vi "GluePattern_Test(SubVI).vi"() -> ()   [LabVIEW 2016]
uses:
  C:/Users/Aerotech/Documents/BNL_ThermomechanicalStave/AerotechLibraries/Bin/Aerotech.A3200.dll
  AerotechLibraries/Bin/Aerotech.A3200.dll
  <vilib>/LabVIEW Interface for Arduino/Type Defs/Arduino Resource.ctl
  <vilib>/LabVIEW Interface for Arduino/Type Defs/Board Type.ctl
  <vilib>/LabVIEW Interface for Arduino/Type Defs/Pin Mode.ctl
  <vilib>/Utility/file.llb/Read Delimited Spreadsheet (DBL).vi
  <vilib>/LabVIEW Interface for Arduino/LabVIEW Interface for Arduino.lvlib
panel:
  out "DX [mm]":dbl=4.166666666666667
  out "DY [mm]":dbl=100.0
  in  "Type of Pattern":u16(ring) items=["Dots", "Lines"]
  out "Arduino Resource":T1={"VISA resource"="COM3", "Board Type"=enum."Uno", "Connection Type"=enum."USB / Serial", "Bytes Per Packet (15)"=15}
  in  "Digital I/O Pin":u8=7
  in  "Final Z":dbl=49.0
  out "Final Position":T3={"Final X"=45.83348650187174, "Final Y"=-0.00047053123122535695, "Final Z"=43.999513057466004}
  out "Column":i32=11
  out "Row":i32
  out "error out":errorcluster={"status"=FALSE, "code"=1073676294, "source"="VISA Read in LabVIEW Interface for Arduino.lvlib:Send Receive.vi->LabVIEW Interface for Arduino.lvlib:Digital Write Pin.vi->GluePattern_Test(SubVI).vi"}
  in  "Home?":bool
  out "XYZ Stage Control":refnum<k24>
  in  "File to be processed- Dots":path=path "C:/Users/Aerotech/Documents/BNL_ThermomechanicalStave/1_ModulePlacement/1_GluePatterning/LabVIEW_gluepattern_arraytest.csv"
  in  "Axis Speeds":T4={"vX [mm]"=15.0, "vY [mm]"=15.0, "vZ [mm] "=15.0}
  in  "Go to \ncoordinates":T5={"X [mm]"=0.0, "Y [mm]"=0.0, "Z [mm] "=44.0}
  out "DX[s]":dbl=0.2777777777777778 format="%#_2g"
  out "DY [s]":dbl=6.666666666666667 format="%#_2g"
  in  "Module width [mm]":dbl=50.0
  in  "Module length [mm]":dbl=100.0
  out "INPUT : Dot":bool[][](array[boolean])=[[TRUE, FALSE, TRUE, FALSE, TRUE, FALSE, TRUE, FALSE, TRUE, FALSE, TRUE, FALSE]]
  in  "Duration of glue \ndispensing [s]":dbl=0.25
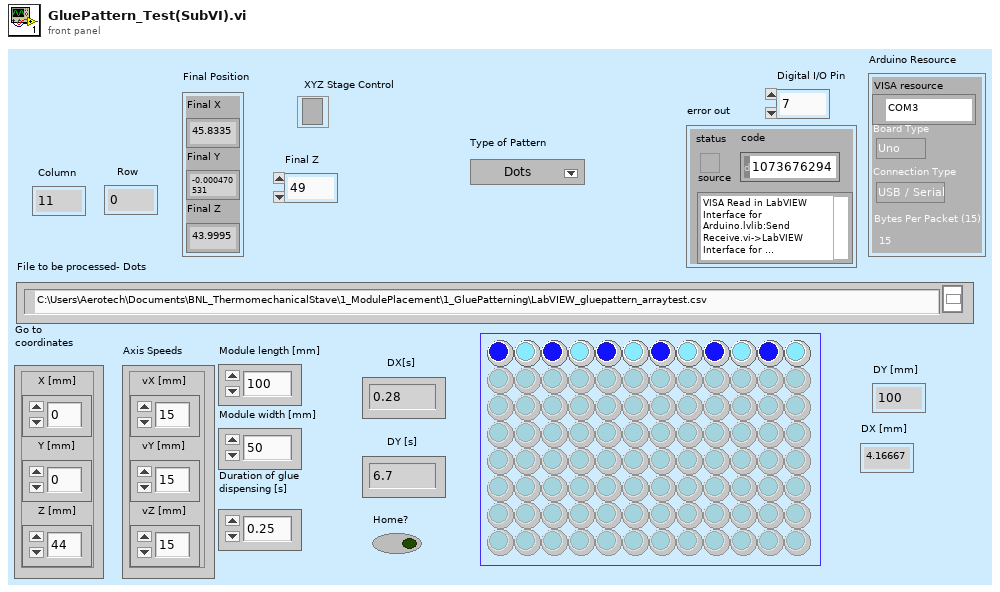
[diagram p1: front panel]
types:
  T1 = typedef "LabVIEW Interface for Arduino.lvlib/Arduino Resource.ctl" = cluster{"VISA resource":refnum<visa-resource-name>, "Board Type":T2, "Connection Type":enum8{"USB / Serial"}, "Bytes Per Packet (15)":u8}
  T2 = typedef "LabVIEW Interface for Arduino.lvlib/Board Type.ctl" = enum16{"Uno", "Dimuelanove w/Atmega 328", "Mega 2560"}
  T3 = cluster{"Final X":dbl, "Final Y":dbl, "Final Z":dbl}
  T4 = cluster{"vX [mm]":dbl, "vY [mm]":dbl, "vZ [mm] ":dbl}
  T5 = cluster{"X [mm]":dbl, "Y [mm]":dbl, "Z [mm] ":dbl}
  T6 = typedef "LabVIEW Interface for Arduino.lvlib/Pin Mode.ctl" = enum8{"Input", "Output"}
  T7 = cluster{"X [mm]":dbl, "Y [mm]":dbl, "Z [mm]":dbl}
  T8 = cluster{"X Position Feedback":dbl, "Y Position Feedback":dbl, "Z Position Feedback":dbl}
  T9 = cluster{"Final X":dbl, "Final Y":dbl, "Z [mm] ":dbl}
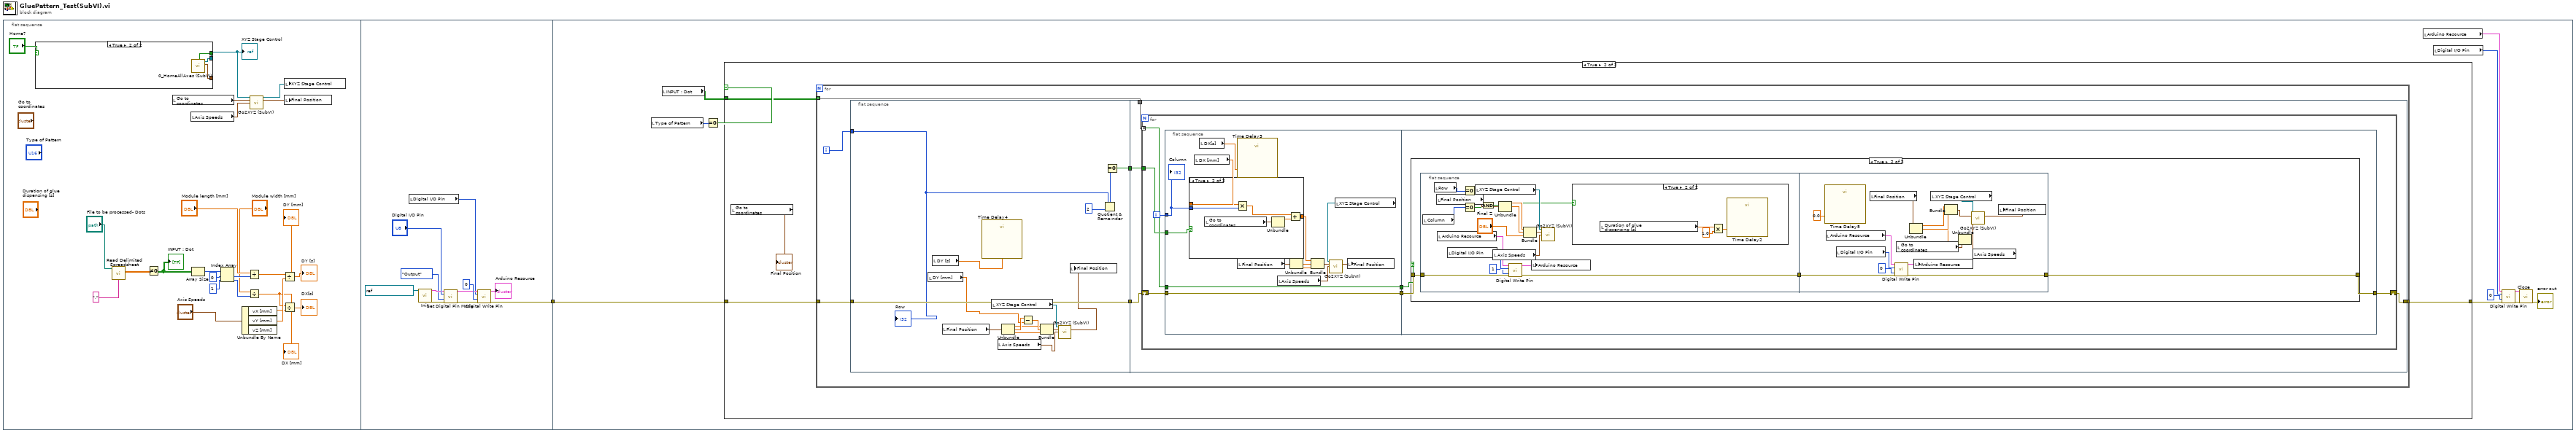
[diagram p0: block diagram]
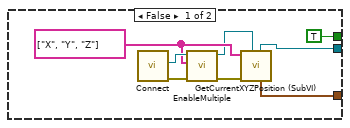
[diagram p2: hidden frame]
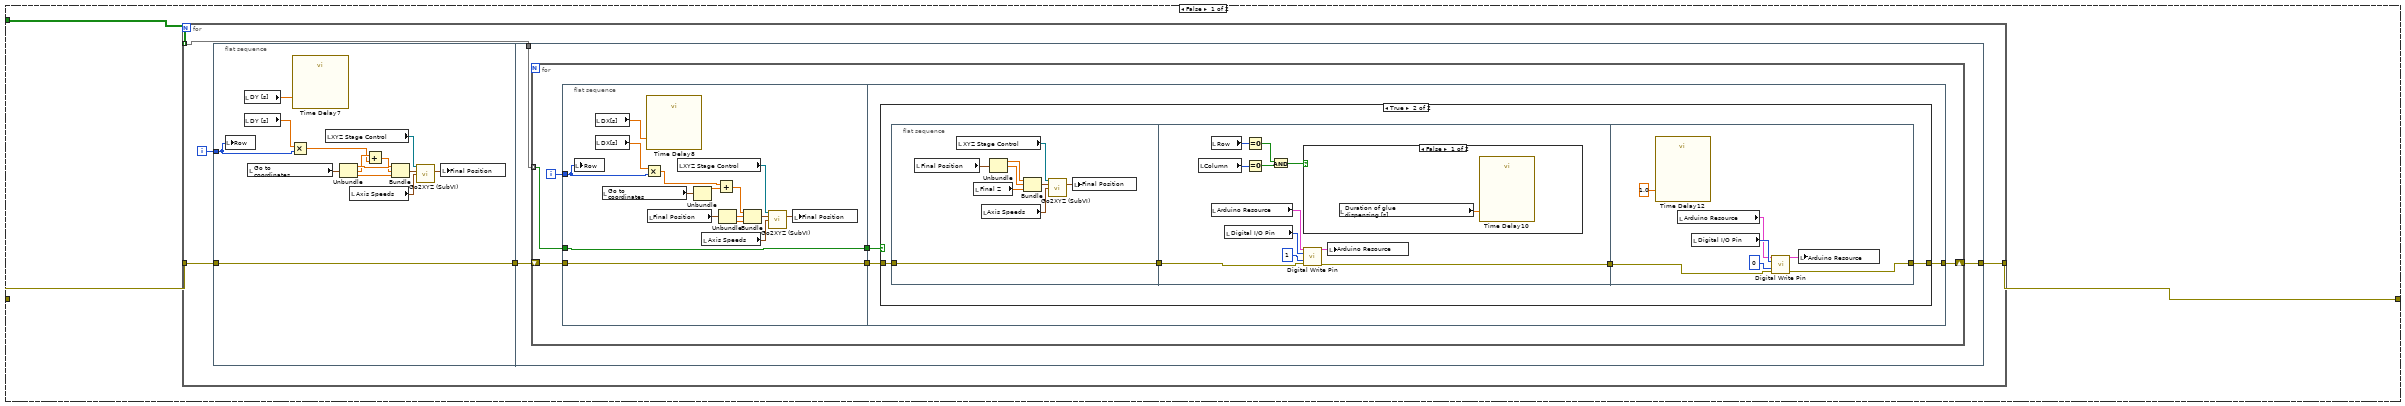
[diagram p3: hidden frame]
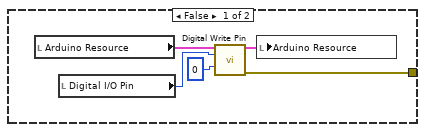
[diagram p4: hidden frame]
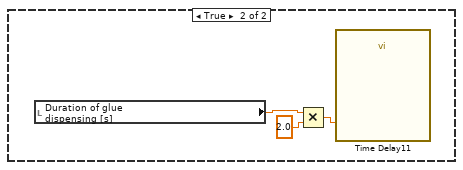
[diagram p5: hidden frame]
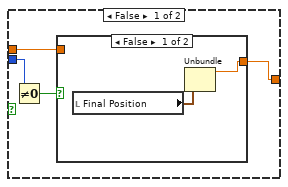
[diagram p6: hidden frame]
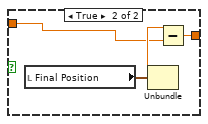
[diagram p7: hidden frame]
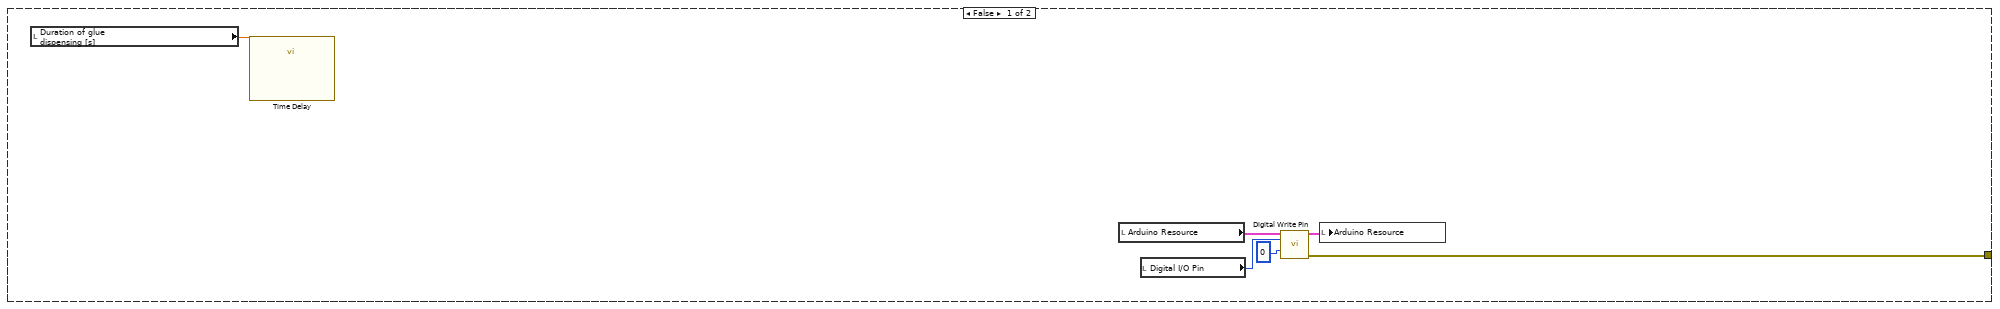
[diagram p8: hidden frame]
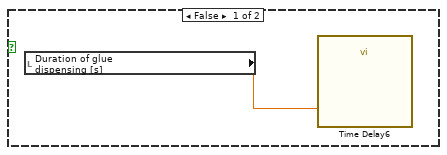
[diagram p9: hidden frame]
diagram:
  n1 = flat-sequence {
    tunnel: [w39] -> w1
    tunnel: w1 -> [w50]
    frame #0 {
      n2 = case shown="True" "Home?" {
        tunnel: [w26 w36] -> _
        tunnel: [TRUE ("completed") w35] -> _
        tunnel: [w28 w34] -> w7
        frame False {
          w30 = string[] ["X", "Y", "Z"] ("Axes Names")
          n3 = call "Connect.vi"() -> ("error out"=w32:errorcluster, "controller"=w31:refnum<k24>)  [unwired: 10 in]
          n4 = call "EnableMultiple.vi"("error in (no error)"=w32, "axis names"=w30, "controller in"=w31) -> ("error out"=w33:errorcluster, "controller out"=w29:refnum<k24>)  [unwired: 7 in]
          n5 = call "GetCurrentXYZPosition (SubVI).vi"(".NET Refnum in - Device"=w29, "error in (no error)"=w33, "Axes Names"=w30) -> ("Current stage position"=w26:T7, ".NET Refnum out  - Device"=w28:refnum<k24>)  [unwired: 3 in, 4 out]
        }
        frame True {
          n6 = call "0_HomeAllAxes (SubVI).vi"() -> ("Homed coordinates"=w36:T8, "controller out"=w34:refnum<k24>, "completed"=w35:bool)  [unwired: 8 in, 1 out]
        }
      }
      "XYZ Stage Control" <- w7
      n7 = call-poly <vilib>:"Read Delimited Spreadsheet.vi"("file path (dialog if empty)"="File to be processed- Dots", "delimiter (\\t)"="," ("delimiter (\\t)")) -> ("all rows"=w24:dbl[][])  [unwired: 8 in, 5 out]
      n8 = Not Equal To 0?(x=w24) -> (x != 0?=w8:bool[][])
      "INPUT : Dot" <- w8
      n9 = local read "Go to \ncoordinates"() -> (w2:T5)
      n10 = local read "Axis Speeds"() -> (w4:T4)
      n11 = Array Size(array=w8) -> (size(s)=w23:i32[])
      n12 = Index Array(array=w23, index #1=0 ("index"), index #2=1 ("index")) -> (element #1=w19:i32, element #2=w18:i32)
      n13 = Unbundle By Name("Axis Speeds") -> ("vX [mm]"=w14:dbl, "vY [mm]"=w15:dbl)  [unwired: 1 out]
      n14 = Divide(x="Module length [mm]", y=w19) -> (x/y=w16:dbl)
      "DY [mm]" <- w16
      n15 = Divide(x="Module width [mm]", y=w18) -> (x/y=w13:dbl)
      "DX [mm]" <- w13
      n16 = call "Go2XYZ (SubVI).vi"(".NET Refnum in"=w7, "Go to Coordinates"=w2, "Axis Speeds"=w4) -> (".NET Refnum out"=w3:refnum<k24>, "Final Position"=w5:T3)  [unwired: 8 in, 3 out]
      n17 = Divide(x=w16, y=w15) -> (x/y=→"DY [s]":dbl)
      n18 = Divide(x=w13, y=w14) -> (x/y=→"DX[s]":dbl)
      n19 = local write "XYZ Stage Control"(w3) -> ()
      n20 = local write "Final Position"(w5) -> ()
    }
    frame #1 {
      n21 = local read "Digital I/O Pin"() -> (w37:u8)
      n22 = call <vilib>:"Init.vi"("VISA resource"=refnum<visa-resource-name> "COM3") -> ("Arduino Resource"=w42:T1, "error out"=w40:errorcluster)  [unwired: 17 in]
      n23 = call <vilib>:"Set Digital Pin Mode.vi"("Arduino Resource"=w42, "Digital I/O Pin"="Digital I/O Pin", "Pin Mode (Input)"=Pin_Mode."Output", "error in"=w40) -> ("Arduino Resource"=w44:T1, "error out"=w45:errorcluster)  [unwired: 10 in]
      n24 = call <vilib>:"Digital Write Pin.vi"("Arduino Resource"=w44, "Digital I/O Pin (0)"=w37, "Value (0)"=u8 0, "error in"=w45) -> ("Arduino Resource"=→"Arduino Resource":T1, "error out"=w39:errorcluster)  [unwired: 10 in]
    }
    frame #2 {
      n25 = local read "Type of Pattern"() -> (w49:u16)
      n26 = local read "INPUT : Dot"() -> (w54:bool[][])
      n27 = Equal To 0?(x=w49) -> (x = 0?=w48:bool)
      n28 = case shown="True" w48 {
        tunnel: w54 -> [w59 w152]
        tunnel: [w60 w151] -> w51
        tunnel: w50 -> [w61 w150]
        frame False {
          n29 = for {
            tunnel: w59 -> [w62] mode=indexing
            tunnel: [w65] -> w60
            tunnel: w61 -> [w63]
            i -> [w66]
            n30 = flat-sequence {
              tunnel: w66 -> [w67]
              tunnel: [w69] -> w64
              tunnel: w63 -> [w69]
              tunnel: w62 -> [w83]
              tunnel: [w82] -> w65
              tunnel: w64 -> [w81]
              frame #0 {
                n31 = local write "Row"(w67) -> ()
                n32 = local read "DY [s]"() -> (w80:dbl)
                n33 = local read "DY [s]"() -> (w77:dbl)
                n34 = local read "Go to \ncoordinates"() -> (w75:T5)
                n35 = Multiply(x=w77, y=w67) -> (x*y=w71:dbl)
                n36 = call "Time Delay7"("Delay Time (s)"=w80) -> ()  [unwired: 10 in, 1 out]
                n37 = local read "XYZ Stage Control"() -> (w78:refnum<k24>)
                n38 = Unbundle(w75) -> ("X [mm]"=w74:dbl, "Y [mm]"=w72:dbl, "Z [mm]"=w73:dbl)
                n39 = local read "Axis Speeds"() -> (w79:T4)
                n40 = Add(x=w72, y=w71) -> (x+y=w70:dbl)
                n41 = Bundle("X [mm]"=w74, w70, "Z [mm]"=w73) -> (w76:cluster{"X [mm]":dbl, dbl, "Z [mm] ":dbl})  [unwired: 1 in]
                n42 = call "Go2XYZ (SubVI).vi"(".NET Refnum in"=w78, "Go to Coordinates"=w76, "Axis Speeds"=w79) -> ("Final Position"=w68:T3)  [unwired: 8 in, 4 out]
                n43 = local write "Final Position"(w68) -> ()
              }
              frame #1 {
                n44 = for {
                  shift-right: [w84] -> w82
                  shift-left: w81 -> [w88]
                  tunnel: w83 -> [w85] mode=indexing
                  i -> [w89]
                  n45 = flat-sequence {
                    tunnel: w89 -> [w91]
                    tunnel: w88 -> [w101]
                    tunnel: [w101] -> w87
                    tunnel: [w100] -> w86
                    tunnel: w85 -> [w100]
                    tunnel: w87 -> [w108]
                    tunnel: w86 -> [w106]
                    tunnel: [w107] -> w84
                    frame #0 {
                      n46 = local write "Row"(w91) -> ()
                      n47 = local read "DX[s]"() -> (w102:dbl)
                      n48 = local read "DX[s]"() -> (w103:dbl)
                      n49 = local read "Go to \ncoordinates"() -> (w95:T5)
                      n50 = Multiply(x=w103, y=w91) -> (x*y=w94:dbl)
                      n51 = call "Time Delay8"("Delay Time (s)"=w102) -> ()  [unwired: 10 in, 1 out]
                      n52 = local read "Final Position"() -> (w90:T3)
                      n53 = local read "XYZ Stage Control"() -> (w104:refnum<k24>)
                      n54 = Unbundle(w95) -> ("X [mm]"=w93:dbl)  [unwired: 2 out]
                      n55 = local read "Axis Speeds"() -> (w105:T4)
                      n56 = Add(x=w94, y=w93) -> (x+y=w92:dbl)
                      n57 = Unbundle(w90) -> ("Final Y"=w99:dbl, "Final Z"=w96:dbl)  [unwired: 1 out]
                      n58 = Bundle(w92, "Final Y"=w99, "Final Z"=w96) -> (w97:cluster{dbl, "Final Y":dbl, "Final Z":dbl})  [unwired: 1 in]
                      n59 = call "Go2XYZ (SubVI).vi"(".NET Refnum in"=w104, "Go to Coordinates"=w97, "Axis Speeds"=w105) -> ("Final Position"=w98:T3)  [unwired: 8 in, 4 out]
                      n60 = local write "Final Position"(w98) -> ()
                    }
                    frame #1 {
                      n61 = case shown="True" w106 {
                        tunnel: [w112 w115] -> w107
                        tunnel: w108 -> [_ w116]
                        frame False {
                          n62 = local read "Arduino Resource"() -> (w111:T1)
                          n63 = local read "Digital I/O Pin"() -> (w110:u8)
                          n64 = call <vilib>:"Digital Write Pin.vi"("Arduino Resource"=w111, "Digital I/O Pin (0)"=w110, "Value (0)"=u8 0) -> ("Arduino Resource"=w109:T1, "error out"=w112:errorcluster)  [unwired: 11 in]
                          n65 = local write "Arduino Resource"(w109) -> ()
                        }
                        frame True {
                          n66 = flat-sequence {
                            tunnel: [w124] -> w117
                            tunnel: w116 -> [w124]
                            tunnel: w117 -> [w132]
                            tunnel: [w136] -> w114
                            tunnel: [w142] -> w115
                            tunnel: w114 -> [w143]
                            frame #0 {
                              n67 = local read "Final Position"() -> (w122:T3)
                              n68 = local read "XYZ Stage Control"() -> (w125:refnum<k24>)
                              n69 = local read "Final Z"() -> (w119:dbl)
                              n70 = local read "Axis Speeds"() -> (w126:T4)
                              n71 = Unbundle(w122) -> ("Final X"=w121:dbl, "Final Y"=w120:dbl)  [unwired: 1 out]
                              n72 = Bundle("Final X"=w121, "Final Y"=w120, "Final Z"=w119) -> (w123:T3)  [unwired: 1 in]
                              n73 = call "Go2XYZ (SubVI).vi"(".NET Refnum in"=w125, "Go to Coordinates"=w123, "Axis Speeds"=w126) -> ("Final Position"=w118:T3)  [unwired: 8 in, 4 out]
                              n74 = local write "Final Position"(w118) -> ()
                            }
                            frame #1 {
                              n75 = local read "Column"() -> (w129:i32)
                              n76 = local read "Row"() -> (w131:i32)
                              n77 = local read "Arduino Resource"() -> (w135:T1)
                              n78 = local read "Digital I/O Pin"() -> (w134:u8)
                              n79 = Equal To 0?(x=w131) -> (x = 0?=w130:bool)
                              n80 = Equal To 0?(x=w129) -> (x = 0?=w128:bool)
                              n81 = And(x=w130, y=w128) -> (x .and. y?=w127:bool)
                              n82 = case shown="False" w127 {
                                frame False {
                                n83 = local read "Duration of glue \ndispensing [s]"() -> (w138:dbl)
                                n84 = call "Time Delay10"("Delay Time (s)"=w138) -> ()  [unwired: 10 in, 1 out]
                                }
                                frame True {
                                n85 = local read "Duration of glue \ndispensing [s]"() -> (w140:dbl)
                                n86 = Multiply(x=w140, y=2.0) -> (x*y=w139:dbl)
                                n87 = call "Time Delay11"("Delay Time (s)"=w139) -> ()  [unwired: 10 in, 1 out]
                                }
                              }
                              n88 = call <vilib>:"Digital Write Pin.vi"("Arduino Resource"=w135, "Digital I/O Pin (0)"=w134, "Value (0)"=u8 1, "error in"=w132) -> ("Arduino Resource"=w133:T1, "error out"=w136:errorcluster)  [unwired: 10 in]
                              n89 = local write "Arduino Resource"(w133) -> ()
                            }
                            frame #2 {
                              n90 = call "Time Delay12"("Delay Time (s)"=1.0) -> ()  [unwired: 10 in, 1 out]
                              n91 = local read "Arduino Resource"() -> (w144:T1)
                              n92 = local read "Digital I/O Pin"() -> (w145:u8)
                              n93 = call <vilib>:"Digital Write Pin.vi"("Arduino Resource"=w144, "Digital I/O Pin (0)"=w145, "Value (0)"=u8 0, "error in"=w143) -> ("Arduino Resource"=w147:T1, "error out"=w142:errorcluster)  [unwired: 10 in]
                              n94 = local write "Arduino Resource"(w147) -> ()
                            }
                          }
                        }
                      }
                    }
                  }
                }
              }
            }
          }
        }
        frame True {
          n95 = local read "Go to \ncoordinates"() -> (→"Final Position":T5)
          n96 = for {
            tunnel: w152 -> [w157] mode=indexing
            tunnel: [w156] -> w151
            tunnel: w150 -> [w154]
            i -> [w158]
            n97 = flat-sequence {
              tunnel: w158 -> [w162]
              tunnel: [w174] -> w155
              tunnel: w154 -> [w174]
              tunnel: [w159] -> w153
              tunnel: w157 -> [w178]
              tunnel: [w177] -> w156
              tunnel: w155 -> [w176]
              tunnel: w153 -> [w175]
              frame #0 {
                n98 = local read "DY [mm]"() -> (w163:dbl)
                n99 = local read "DY [s]"() -> (w165:dbl)
                n100 = local read "Final Position"() -> (w168:T3)
                n101 = call "Time Delay4"("Delay Time (s)"=w165) -> ()  [unwired: 10 in, 1 out]
                n102 = local read "XYZ Stage Control"() -> (w166:refnum<k24>)
                n103 = local read "Axis Speeds"() -> (w173:T4)
                n104 = Unbundle(w168) -> ("Final X"=w169:dbl, "Final Y"=w171:dbl, "Final Z"=w170:dbl)
                n105 = Subtract(x=w171, y=w163) -> (x-y=w172:dbl)
                n106 = Bundle("Final X"=w169, w172, "Final Z"=w170) -> (w167:cluster{"Final X":dbl, dbl, "Final Z":dbl})  [unwired: 1 in]
                n107 = call "Go2XYZ (SubVI).vi"(".NET Refnum in"=w166, "Go to Coordinates"=w167, "Axis Speeds"=w173) -> ("Final Position"=w164:T3)  [unwired: 8 in, 4 out]
                n108 = local write "Final Position"(w164) -> ()
                n109 = Quotient & Remainder(x=w162, y=2) -> (x-y*floor(x/y)=w160:i32)  [unwired: 1 out]
                n110 = Equal To 0?(x=w160) -> (x = 0?=w159:bool)
                "Row" <- w162
              }
              frame #1 {
                n111 = for {
                  shift-right: [w180] -> w177
                  shift-left: w176 -> [w184]
                  tunnel: w178 -> [w181] mode=indexing
                  tunnel: w175 -> [w179]
                  i -> [w185]
                  n112 = flat-sequence {
                    tunnel: w185 -> [w196]
                    tunnel: w184 -> [w194]
                    tunnel: [w194] -> w183
                    tunnel: [w193] -> w182
                    tunnel: w181 -> [w193]
                    tunnel: w179 -> [w186]
                    tunnel: w183 -> [w218]
                    tunnel: w182 -> [w216]
                    tunnel: [w217] -> w180
                    frame #0 {
                      n113 = local read "DX [mm]"() -> (w197:dbl)
                      n114 = case shown="True" w186 {
                        tunnel: w197 -> [w203 w215]
                        tunnel: w196 -> [w200 w214]
                        tunnel: [w202 w210] -> w187
                        frame False {
                          n115 = Not Equal To 0?(x=w200) -> (x != 0?=w201:bool)
                          n116 = case shown="False" w201 {
                            tunnel: w203 -> [_ w207]
                            tunnel: [w204 w206] -> w202
                            frame False {
                              n117 = local read "Final Position"() -> (w205:T3)
                              n118 = Unbundle(w205) -> ("Final X"=w204:dbl)  [unwired: 2 out]
                            }
                            frame True {
                              n119 = local read "Final Position"() -> (w209:T3)
                              n120 = Unbundle(w209) -> ("Final X"=w208:dbl)  [unwired: 2 out]
                              n121 = Subtract(x=w208, y=w207) -> (x-y=w206:dbl)
                            }
                          }
                        }
                        frame True {
                          n122 = local read "Go to \ncoordinates"() -> (w213:T5)
                          n123 = Multiply(x=w215, y=w214) -> (x*y=w212:dbl)
                          n124 = Unbundle(w213) -> ("X [mm]"=w211:dbl)  [unwired: 2 out]
                          n125 = Add(x=w212, y=w211) -> (x+y=w210:dbl)
                        }
                      }
                      n126 = local read "DX[s]"() -> (w195:dbl)
                      n127 = call "Time Delay3"("Delay Time (s)"=w195) -> ()  [unwired: 10 in, 1 out]
                      n128 = local read "Final Position"() -> (w192:T3)
                      n129 = local read "Axis Speeds"() -> (w199:T4)
                      n130 = Unbundle(w192) -> ("Final Y"=w191:dbl, "Final Z"=w188:dbl)  [unwired: 1 out]
                      n131 = Bundle("Final X"=w187, "Final Y"=w191, "Final Z"=w188) -> (w189:T3)  [unwired: 1 in]
                      n132 = local read "XYZ Stage Control"() -> (w198:refnum<k24>)
                      n133 = call "Go2XYZ (SubVI).vi"(".NET Refnum in"=w198, "Go to Coordinates"=w189, "Axis Speeds"=w199) -> ("Final Position"=w190:T3)  [unwired: 8 in, 4 out]
                      n134 = local write "Final Position"(w190) -> ()
                      "Column" <- w196
                    }
                    frame #1 {
                      n135 = case shown="True" w216 {
                        tunnel: [w223 w226] -> w217
                        tunnel: w218 -> [_ w227]
                        frame False {
                          n136 = local read "Duration of glue \ndispensing [s]"() -> (w222:dbl)
                          n137 = call "Time Delay"("Delay Time (s)"=w222) -> ()  [unwired: 10 in, 1 out]
                          n138 = local read "Arduino Resource"() -> (w221:T1)
                          n139 = local read "Digital I/O Pin"() -> (w220:u8)
                          n140 = call <vilib>:"Digital Write Pin.vi"("Arduino Resource"=w221, "Digital I/O Pin (0)"=w220, "Value (0)"=u8 0) -> ("Arduino Resource"=w219:T1, "error out"=w223:errorcluster)  [unwired: 11 in]
                          n141 = local write "Arduino Resource"(w219) -> ()
                        }
                        frame True {
                          n142 = flat-sequence {
                            tunnel: [w241] -> w225
                            tunnel: w227 -> [w241]
                            tunnel: [w258] -> w226
                            tunnel: w225 -> [w259]
                            frame #0 {
                              n143 = local read "Column"() -> (w234:i32)
                              n144 = local read "Row"() -> (w232:i32)
                              n145 = local read "Final Position"() -> (w239:T3)
                              n146 = local read "Arduino Resource"() -> (w229:T1)
                              n147 = local read "Digital I/O Pin"() -> (w230:u8)
                              n148 = Equal To 0?(x=w232) -> (x = 0?=w233:bool)
                              n149 = Equal To 0?(x=w234) -> (x = 0?=w235:bool)
                              n150 = local read "XYZ Stage Control"() -> (w242:refnum<k24>)
                              n151 = And(x=w233, y=w235) -> (x .and. y?=w236:bool)
                              n152 = local read "Axis Speeds"() -> (w243:T4)
                              n153 = Unbundle(w239) -> ("Final X"=w238:dbl, "Final Y"=w237:dbl)  [unwired: 1 out]
                              n154 = call <vilib>:"Digital Write Pin.vi"("Arduino Resource"=w229, "Digital I/O Pin (0)"=w230, "Value (0)"=u8 1) -> ("Arduino Resource"=w231:T1)  [unwired: 11 in, 1 out]
                              n155 = Bundle("Final X"=w238, "Final Y"=w237, "Final Z"="Final Z") -> (w240:T3)  [unwired: 1 in]
                              n156 = local write "Arduino Resource"(w231) -> ()
                              n157 = call "Go2XYZ (SubVI).vi"(".NET Refnum in"=w242, "Go to Coordinates"=w240, "Axis Speeds"=w243) -> ()  [unwired: 8 in, 5 out]
                              n158 = case shown="True" w236 {
                                frame False {
                                n159 = local read "Duration of glue \ndispensing [s]"() -> (w245:dbl)
                                n160 = call "Time Delay6"("Delay Time (s)"=w245) -> ()  [unwired: 10 in, 1 out]
                                }
                                frame True {
                                n161 = local read "Duration of glue \ndispensing [s]"() -> (w247:dbl)
                                n162 = Multiply(x=w247, y=1.0) -> (x*y=w246:dbl)
                                n163 = call "Time Delay2"("Delay Time (s)"=w246) -> ()  [unwired: 10 in, 1 out]
                                }
                              }
                            }
                            frame #1 {
                              n164 = call "Time Delay5"("Delay Time (s)"=0.0) -> ()  [unwired: 10 in, 1 out]
                              n165 = local read "Arduino Resource"() -> (w260:T1)
                              n166 = local read "Digital I/O Pin"() -> (w261:u8)
                              n167 = local read "Final Position"() -> (w257:T3)
                              n168 = call <vilib>:"Digital Write Pin.vi"("Arduino Resource"=w260, "Digital I/O Pin (0)"=w261, "Value (0)"=u8 0, "error in"=w259) -> ("Arduino Resource"=w263:T1, "error out"=w258:errorcluster)  [unwired: 10 in]
                              n169 = local read "Go to \ncoordinates"() -> (w256:T5)
                              n170 = Unbundle(w257) -> ("Final X"=w255:dbl, "Final Y"=w254:dbl)  [unwired: 1 out]
                              n171 = local write "Arduino Resource"(w263) -> ()
                              n172 = local read "XYZ Stage Control"() -> (w250:refnum<k24>)
                              n173 = Unbundle(w256) -> ("Z [mm]"=w253:dbl)  [unwired: 2 out]
                              n174 = Bundle("Final X"=w255, "Final Y"=w254, "Z [mm]"=w253) -> (w252:T9)  [unwired: 1 in]
                              n175 = local read "Axis Speeds"() -> (w251:T4)
                              n176 = call "Go2XYZ (SubVI).vi"(".NET Refnum in"=w250, "Go to Coordinates"=w252, "Axis Speeds"=w251) -> ("Final Position"=w249:T3)  [unwired: 8 in, 4 out]
                              n177 = local write "Final Position"(w249) -> ()
                            }
                          }
                        }
                      }
                    }
                  }
                }
              }
            }
          }
        }
      }
      n178 = local read "Arduino Resource"() -> (w53:T1)
      n179 = local read "Digital I/O Pin"() -> (w52:u8)
      n180 = call <vilib>:"Digital Write Pin.vi"("Arduino Resource"=w53, "Digital I/O Pin (0)"=w52, "Value (0)"=u8 0, "error in"=w51) -> ("Arduino Resource"=w57:T1, "error out"=w58:errorcluster)  [unwired: 10 in]
      n181 = call <vilib>:"Close.vi"("Arduino Resource"=w57, "error in"=w58) -> ("error out"=→"error out":errorcluster)  [unwired: 13 in]
    }
  }
